vi "SVPO RMS Level (1 Ch DBL Array).vi"(6 "restart averaging? (F)":bool, 10 "sampling rate [Hz]":dbl=1.0, 11 "scaled signal [EU]":dbl[](array[numeric])) -> (3 "RMS level":dbl=nan, 4 "duration [s]":dbl)   [LabVIEW 2017, in "SoundVib_VibrationLevel.lvlib"]
doc: "Computes the root-mean-square (RMS) level of scaled time waveform signals and scaled array signals. <B>scaled signal [EU]</B> should have a zero DC component. You can attenuate the DC component with hardware AC-coupling filters and with software high-pass filters. Use this VI on embedded targets that have limited computational resources. Wire data to the <B>scaled signal [EU]</B> input to determine the polymorphic instance to use or manually select the instance."
uses:
  <vilib>/addons/Sound and Vibration/svt_Level/SoundVib_VibrationLevel.lvlib
  <vilib>/Analysis/baseanly.llb/Dot Product.vi
  <vilib>/Analysis/baseanly.llb/Real Dot Product.vi
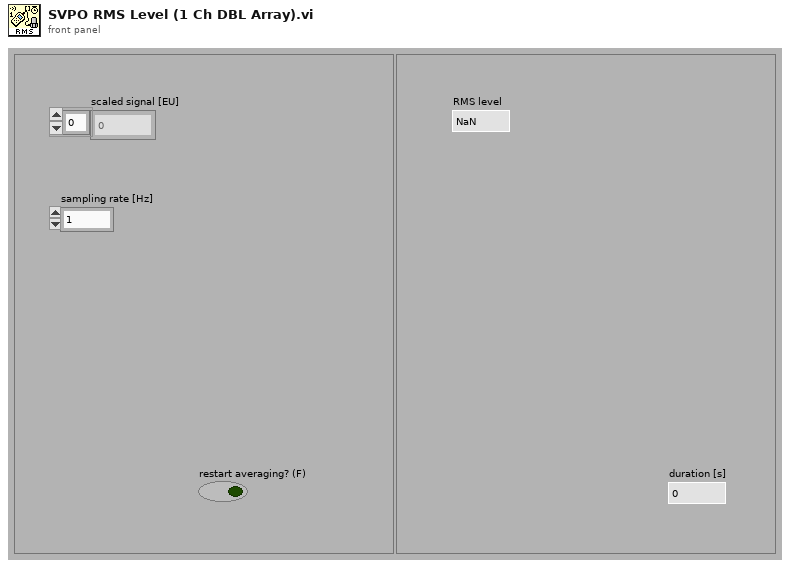
[diagram p1: front panel]
types:
  T1 = typedef "svc_RMS Level State.ctl" = cluster{"Squared Sum":dbl, "Size":u64, "timestamp":timestamp}
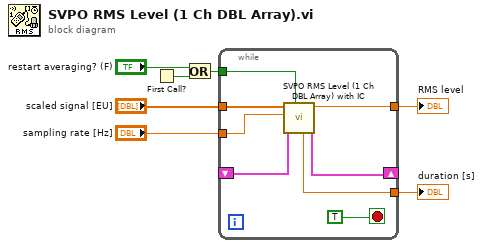
[diagram p0: block diagram]
diagram:
  n1 = First Call?() -> (First Call?: T/F=w7:bool)
  n2 = Or(x="restart averaging? (F)", y=w7) -> (x .or. y?=w5:bool)
  n3 = while {
    tunnel: w5 -> [w11]
    tunnel: "scaled signal [EU]" -> [w14]
    tunnel: [w13] -> w3
    tunnel: [w12] -> w2
    tunnel: "sampling rate [Hz]" -> [w10]
    shift-right: [w9] -> _
    shift-left: _ -> [w8]
    stop <- TRUE stop-if-true
    n4 = call <vilib>:"SVPO RMS Level (1 Ch DBL Array) with IC.vi"("restart averaging? (F)"=w11, "initial conditions"=w8, "sampling rate [Hz]"=w10, "scaled signal [EU]"=w14) -> ("final conditions"=w9:T1, "RMS level"=w13:dbl, "duration [s]"=w12:dbl)  [unwired: 5 in]
  }
  "RMS level" <- w3
  "duration [s]" <- w2
